vi "例程45-主面板.vi"() -> ()   [LabVIEW 2016]
panel:
  in  "弹出子面板":bool
  in  "停止":bool
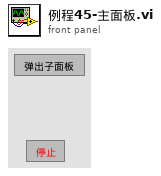
[diagram p1: front panel]
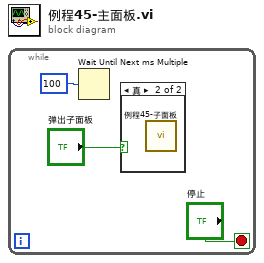
[diagram p0: block diagram]
diagram:
  n1 = while {
    stop <- "停止" stop-if-true
    n2 = Wait Until Next ms Multiple(millisecond multiple=u32 100 ("毫秒倍数")) -> ()  [unwired: 1 out]
    n3 = case shown="真" "弹出子面板" {
      frame False {
      }
      frame True {
        n4 = call "例程45-子面板.vi"() -> ()  [unwired: 12 in]
      }
    }
  }
